vi "dead_lock.vi"() -> ()   [LabVIEW 2019]
panel:
  out "Boolean":bool
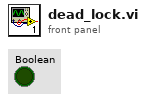
[diagram p1: front panel]
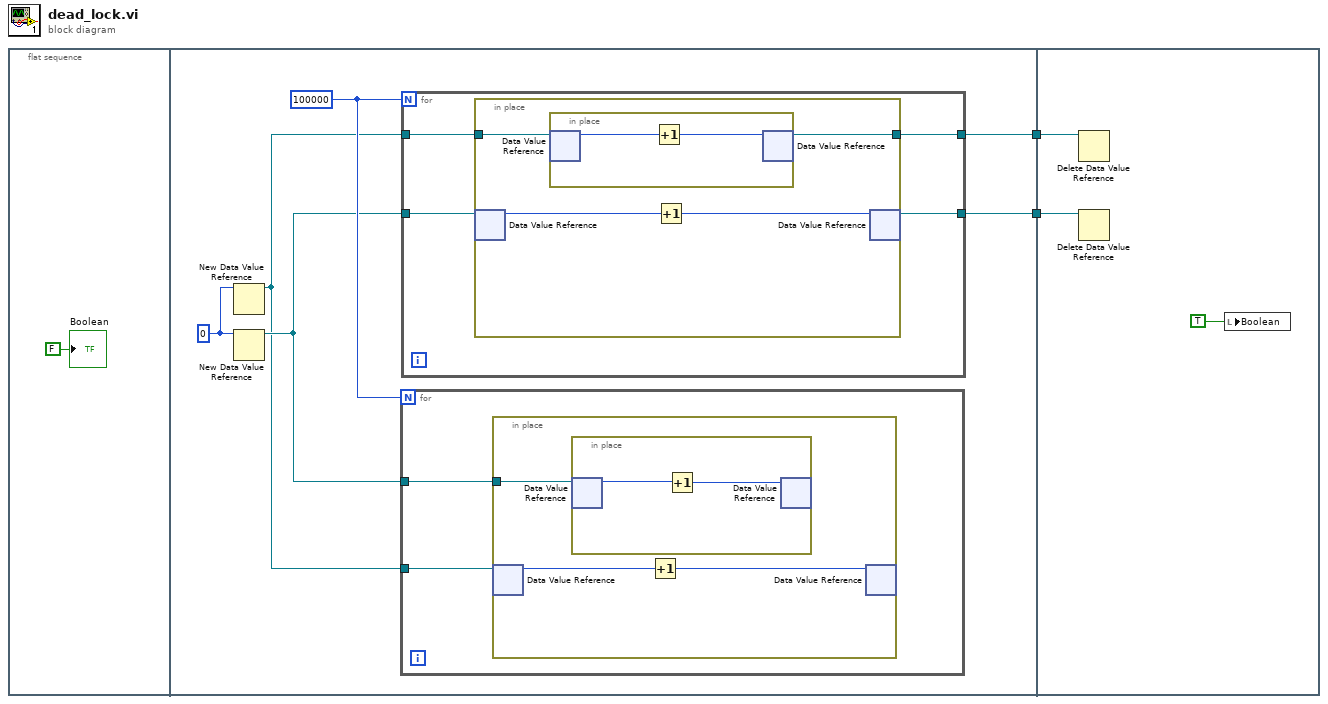
[diagram p0: block diagram]
diagram:
  n1 = flat-sequence {
    tunnel: [w6] -> w2
    tunnel: [w5] -> w1
    tunnel: w2 -> [w28]
    tunnel: w1 -> [w27]
    frame #0 {
      "Boolean" <- FALSE
    }
    frame #1 {
      w9 = 100000
      w7 = 0
      n2 = New Data Value Reference(data value=w7) -> (data value reference=w4:refnum<data-value>)  [unwired: 1 in, 1 out]
      n3 = New Data Value Reference(data value=w7) -> (data value reference=w8:refnum<data-value>)  [unwired: 1 in, 1 out]
      n4 = for {
        N: w9 -> [_]
        tunnel: w8 -> [w10]
        tunnel: w4 -> [w11]
        n5 = in-place {
          in-place-border: w10 -> [w14]
          n6 = in-place-dvr #1(w11) -> (w13:i32)  [unwired: 1 out]
          n7 = in-place {
            n8 = in-place-dvr #2(w14) -> (w16:i32)  [unwired: 1 out]
            n9 = Increment(x=w16) -> (x+1=w15:i32)
            n10 = in-place-dvr #2(w15) -> ()  [unwired: 2 out]
          }
          n11 = Increment(x=w13) -> (x+1=w12:i32)
          n12 = in-place-dvr #1(w12) -> ()  [unwired: 2 out]
        }
      }
      n13 = for {
        N: w9 -> [_]
        tunnel: w8 -> [w18]
        tunnel: w4 -> [w17]
        tunnel: [w20] -> w6
        tunnel: [w19] -> w5
        n14 = in-place {
          in-place-border: w17 -> [w24]
          in-place-border: [w21] -> w20
          n15 = in-place-dvr #3(w18) -> (w23:i32)  [unwired: 1 out]
          n16 = in-place {
            n17 = in-place-dvr #4(w24) -> (w26:i32)  [unwired: 1 out]
            n18 = Increment(x=w26) -> (x+1=w25:i32)
            n19 = in-place-dvr #4(w25) -> (w21:refnum<data-value>)  [unwired: 1 out]
          }
          n20 = Increment(x=w23) -> (x+1=w22:i32)
          n21 = in-place-dvr #3(w22) -> (w19:refnum<data-value>)  [unwired: 1 out]
        }
      }
    }
    frame #2 {
      n22 = Delete Data Value Reference(data value reference=w28) -> ()  [unwired: 1 in, 2 out]
      n23 = Delete Data Value Reference(data value reference=w27) -> ()  [unwired: 1 in, 2 out]
      n24 = local write "Boolean"(TRUE) -> ()
    }
  }
